vi "Load Class.vi"(8 "error in (no error)":errorcluster, 10 "Plugin's IDN":string, 11 "Parent Class":refnum<class "uPluggable.lvclass">) -> (0 "error out":errorcluster, 2 "Plugin":refnum<class "uPluggable.lvclass">)   [LabVIEW 2021, in "uPlug.lvlib" / "uPlugin_Handler.lvclass"]
doc: "Load a plugin by passing in its IDN string and its parent interface/class."
uses:
  uPlugin_Handler.lvclass
  uPluggable/uPluggable.lvclass
  TypeDef_FGV Actions.ctl
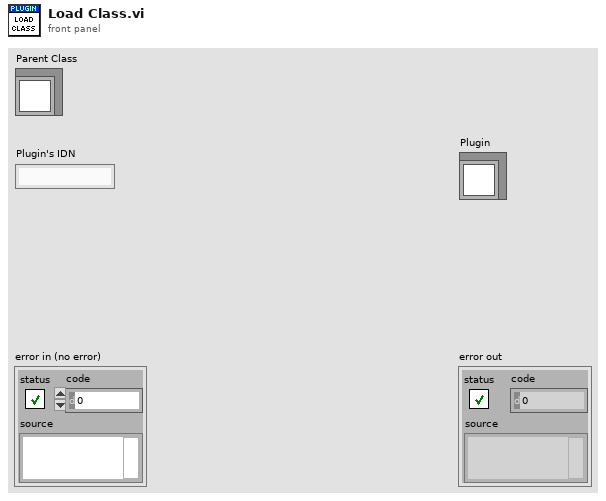
[diagram p1: front panel]
types:
  T1 = typedef "uPlug.lvlib/uPlugin_Handler.lvclass/TypeDef_FGV Actions.ctl" = enum16{"Init", "Load"}
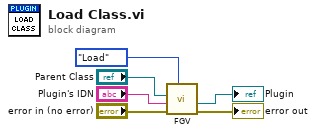
[diagram p0: block diagram]
diagram:
  n1 = call "FGV.vi"("Action"=TypeDef_FGV_Actions."Load", "error in (no error)"="error in (no error)", "Plugin's IDN"="Plugin's IDN", "Parent Class"="Parent Class") -> ("error out"=→"error out":errorcluster, "Plugin"=→"Plugin":refnum<class "uPluggable.lvclass">)  [unwired: 6 in]
